vi "ClassPanel.vi"(8 "error in (no error)":errorcluster caption="entrée d'erreur (pas d'erreur)", 11 "AFG3102C.lvclass":refnum<class "AFG3102C.lvclass">) -> (0 "error out":errorcluster caption="sortie d'erreur", 3 "AFG3102C.lvclass Out":refnum<class "AFG3102C.lvclass">)   [LabVIEW 2019, in "AFG3102C.lvclass"]
uses:
  AFG3102C.lvclass
  C:/Programmes Labview/LabscanV1A/DevicesClass/BaseDevice/BaseDevice.lvclass
  BaseDevice/ClassQueueMess.ctl
  AFG3102C_Func.ctl
  AFG3102C.lvclass/AFG3102C.ctl
  BaseDevice/BaseDevice.lvclass/BaseDevice.ctl
  BaseDevice/Accessor/SetShowInstrNm.vi
  BaseDevice/Accessor/GetClassEvent.vi
  <userlib>/Tektronix AFG 3000 Series/Tektronix AFG 3000 Series.lvlib
panel:
  out "Trig":bool
  in  "Custom Impedance":dbl=400.0
  out "AcqTime":dbl caption="AcqTime(s)" format="%<%M:%S%5u>t"
  in  "Trig and wait":bool
  out "InitPulseLT_us_ch2":dbl=4.0 caption="InitPulseLT(us)" min=0.01 max=1000000000.0 step=0.01
  out "InitPulseHT_us_ch2":dbl=4.0 caption="InitPulseHT(us)" min=0.01 max=1000000000.0 step=0.01
  out "PulsePeriod_us_ch2":dbl=4.0 caption="Pulse Per ch2 (us)" min=0.01 max=1000000000.0 step=0.01
  in  "ForceTrig":bool
  in  "Output En 2":bool caption="Out2 En"
  in  "Out1 En":bool
  out "InitPulseLT_us":dbl=4.0 caption="InitPulseLT(us)" min=0.01 max=1000000000.0 step=0.01
  out "InitPulseHT_us":dbl=4.0 caption="InitPulseHT(us)" min=0.01 max=1000000000.0 step=0.01
  out "PulsePeriod_us":dbl=4.0 caption="Pulse Period (us)" min=0.01 max=1000000000.0 step=0.01
  in  "Con/Disc.":bool
  in  "Tk3102CTab":enum32{"MW Ch1", "Ch2 Laser", "Trig/Func"}(tab)
  in  "BefDel_us":dbl=0.15 caption="BeforeDelay(us)" min=0.0 max=1000000000.0 step=0.001
  in  "HighLevel(V)":dbl=5.0
  in  "LowLevel(V)":dbl
  in  "PLowTime_us":dbl=2.0 caption="Pulse Low\nTime(us)" min=0.01 max=1000000000.0 step=0.01
  in  "PulseCount":i32=30000 caption="Pulse count" min=0 step=1
  in  "BurstDel_us":dbl caption="BurstDelay(us)" min=0.0 max=1000000000.0 step=0.001
  in  "PHighTime_us":dbl=4.0 caption="Pulse High\nTime(us)" min=0.01 max=1000000000.0 step=0.01
  in  "OutputImp":u16(ring) caption="Output Impedance" items=["50 Ohm", "High Impedance", "Customized"]
  in  "AfterPulseDel(us)":dbl=0.1 caption="AfterPulseDelay(us)" min=0.01 max=1000000000.0 step=0.01
  in  "Link Ch":bool=TRUE
  in  "HighLevel(V)ch2":dbl=4.6 caption="HighLevel(V)"
  in  "LowLevel(V)ch2":dbl caption="LowLevel(V)"
  in  "PLowTime_us_ch2":dbl=2.0 caption="Pulse Low\nTime(us)" min=0.01 max=1000000000.0 step=0.01
  in  "PulseCount_ch2":i32=1 caption="Pulse count" min=0 step=1
  in  "PHighTime_us_ch2":dbl=10.0 caption="Pulse High\nTime(us)" min=0.01 max=1000000000.0 step=0.01
  in  "OutputImpch2":u16(ring)=2 caption="Output Impedance" items=["50 Ohm", "High Impedance", "Customized"]
  in  "BurstDel_us_ch2":dbl caption="Burst Delay ch2(us)" min=0.0 max=1000000000.0 step=0.001
  in  "Trigger Source":u16(ring)=1 items=["Internal"=3, "External"=1]
  in  "ExtTrigger Slope":u16(ring)=1 items=["Positive", "Negative"]
  in  "IntTriggRate(s)":dbl=1.0
  in  "Pulse Function":T1(ring)
  in  "Continuous2":bool caption="Continuous"
  out "ControlsNames":string[](array[string])
  in  "MainProgQ":refnum<queue>
  in  "MainProgQEvent":refnum<user-event>
  in  "Acq":bool
  in  "Stop":bool
  out "Init Program":bool
  # "Tek.AFG3102C"
  # "this MUST labeled with class name"
  # "this MUST be present and labeled \"Stop\" and \"Acq\""
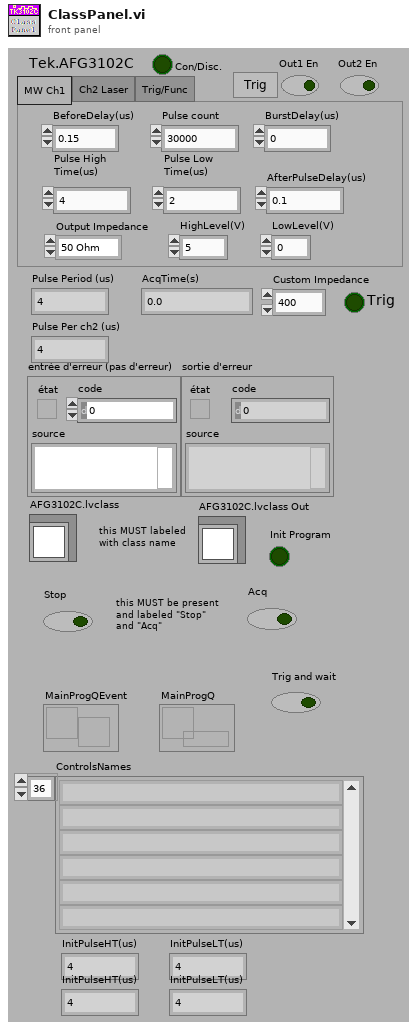
[diagram p1: front panel]
types:
  T1 = enum16{"Rabi", "Ramsey", "Ramsey Ext", "Rabi Ext Laser", "None"}
  T2 = typedef "AFG3102C.lvclass/AFG3102C_Func.ctl" = enum16{"RabiExt (Tau)", "Rabi (Tau)", "RamseyExt (Tau)", "Ramsey (Tau)"}
  T3 = enum16{"Enable", "Disable", "DisAndGrayed", "ReinitToDefVal", "EnumElementsArr"}
  T4 = typedef "ClassQueueMess.ctl" = u16
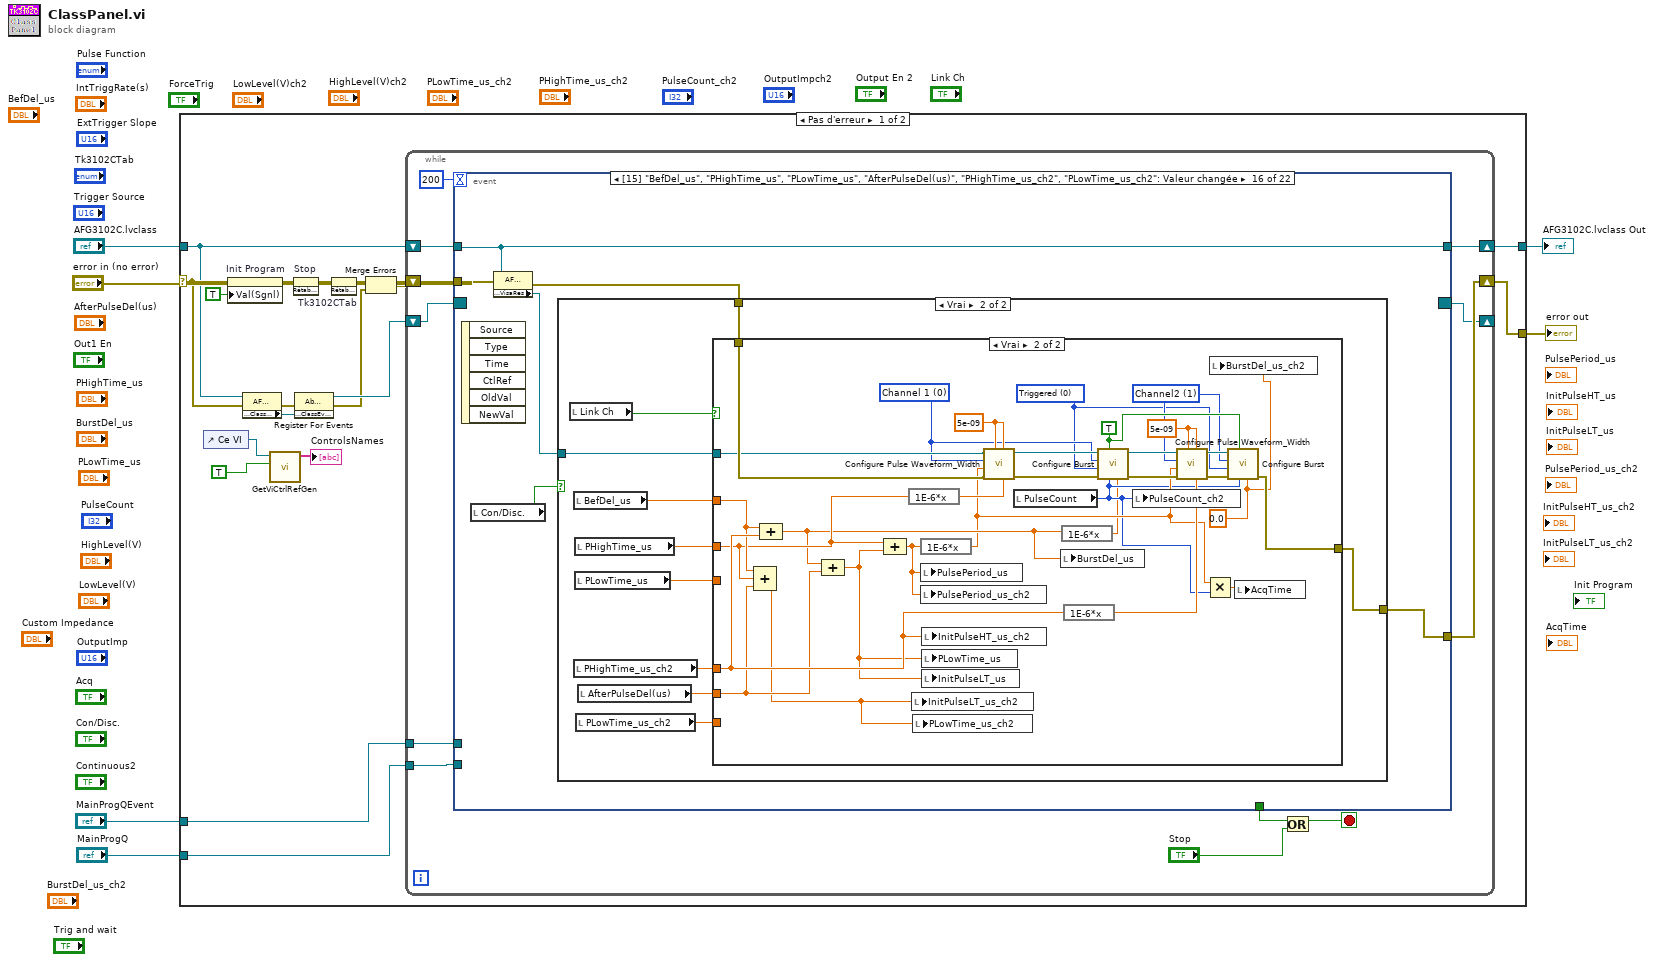
[diagram p0: block diagram]
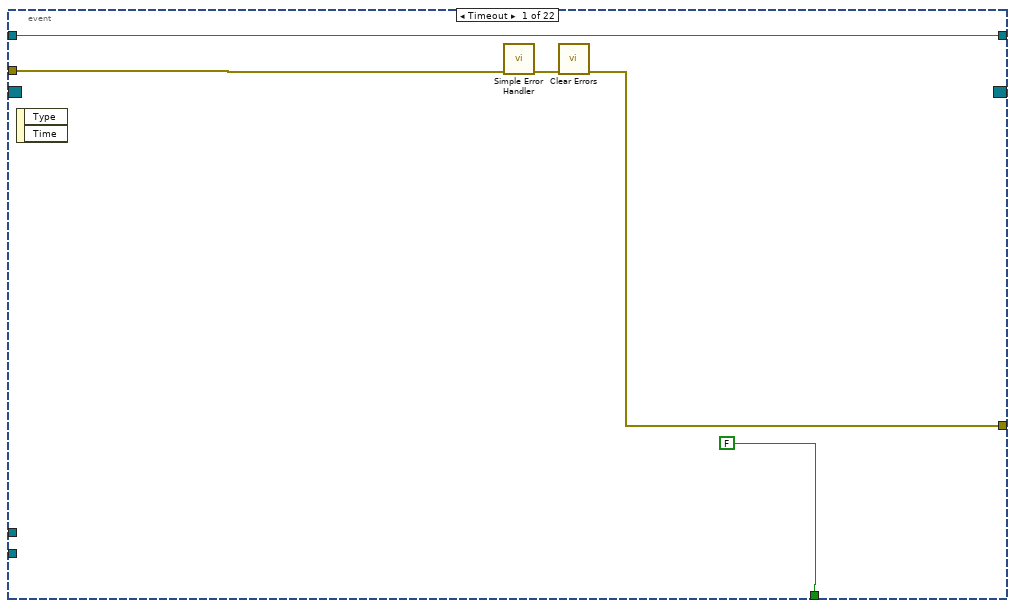
[diagram p2: hidden frame]
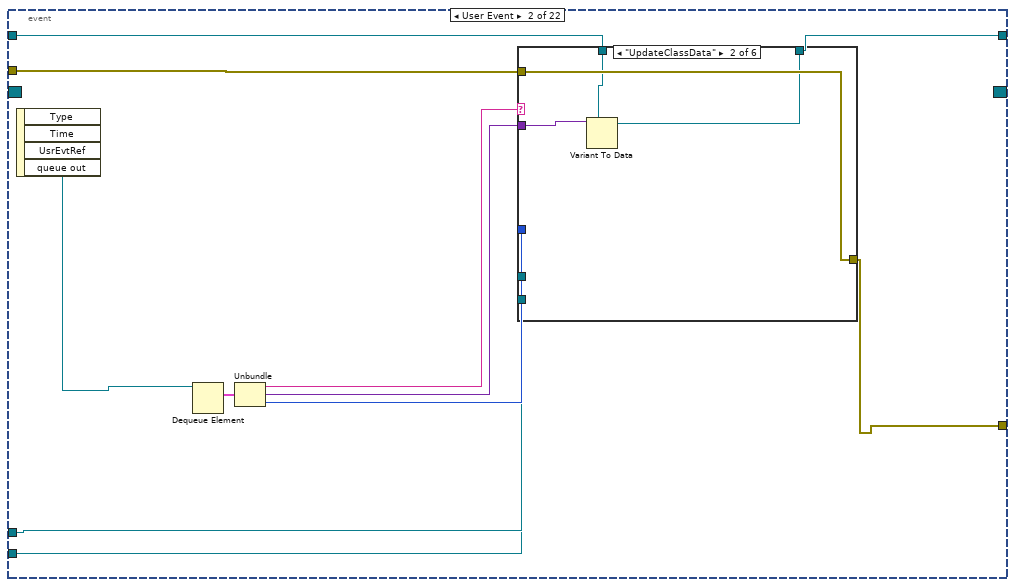
[diagram p3: hidden frame]
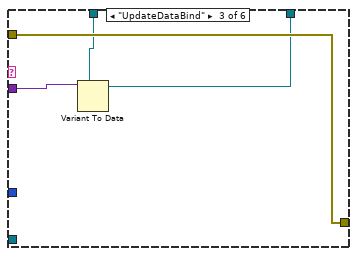
[diagram p5: hidden frame]
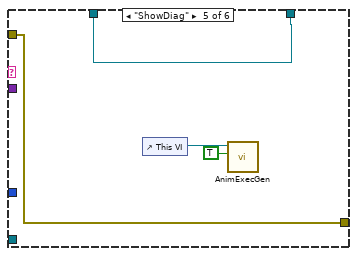
[diagram p7: hidden frame]
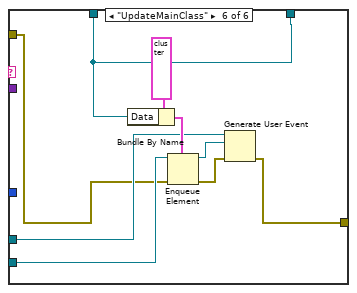
[diagram p8: hidden frame]
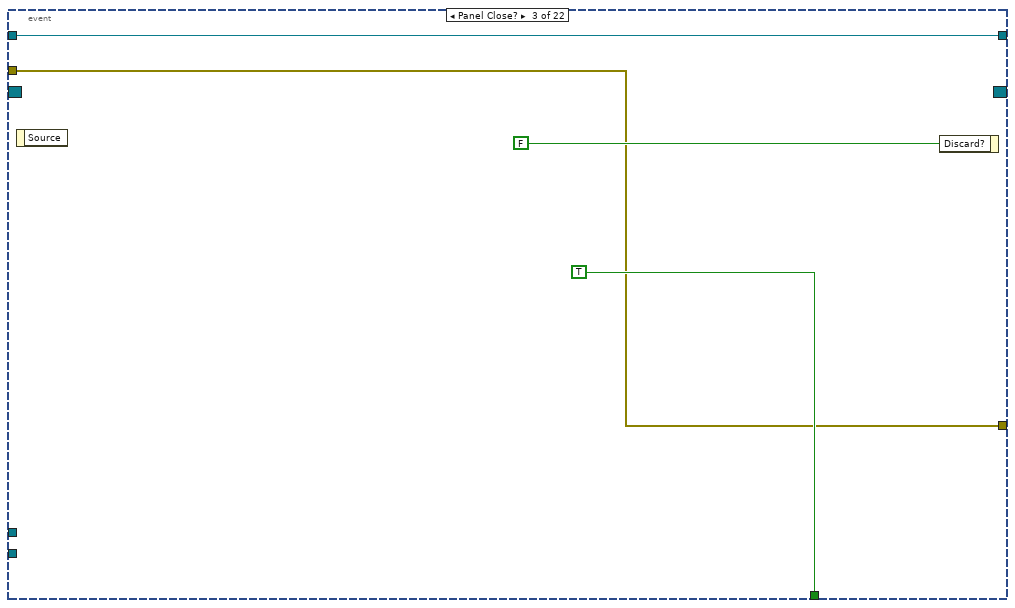
[diagram p9: hidden frame]
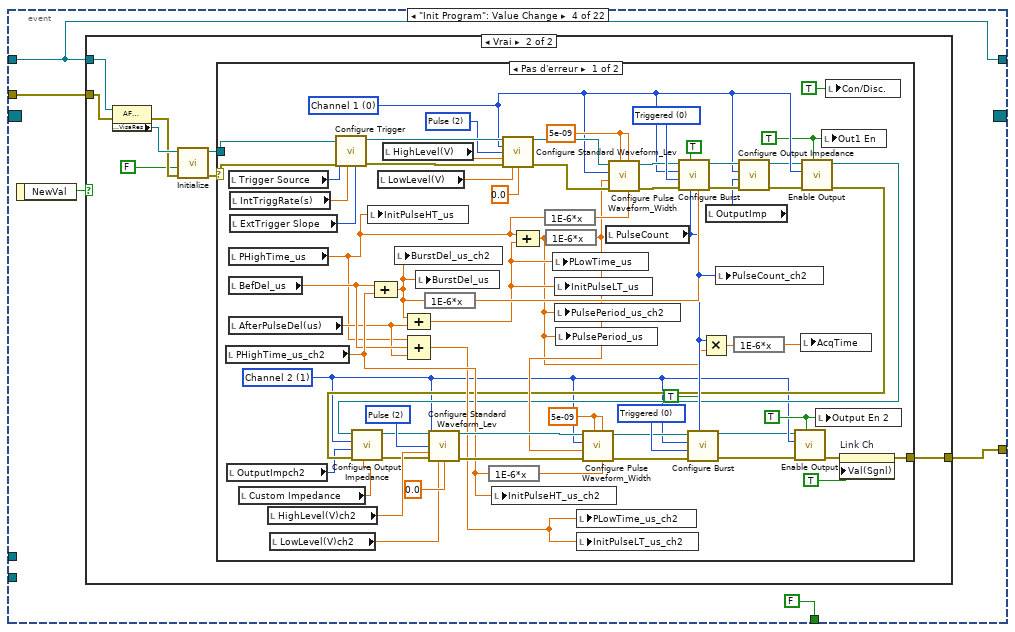
[diagram p10: hidden frame]
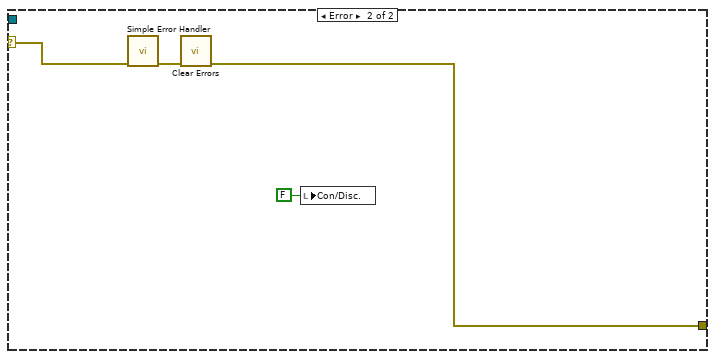
[diagram p12: hidden frame]
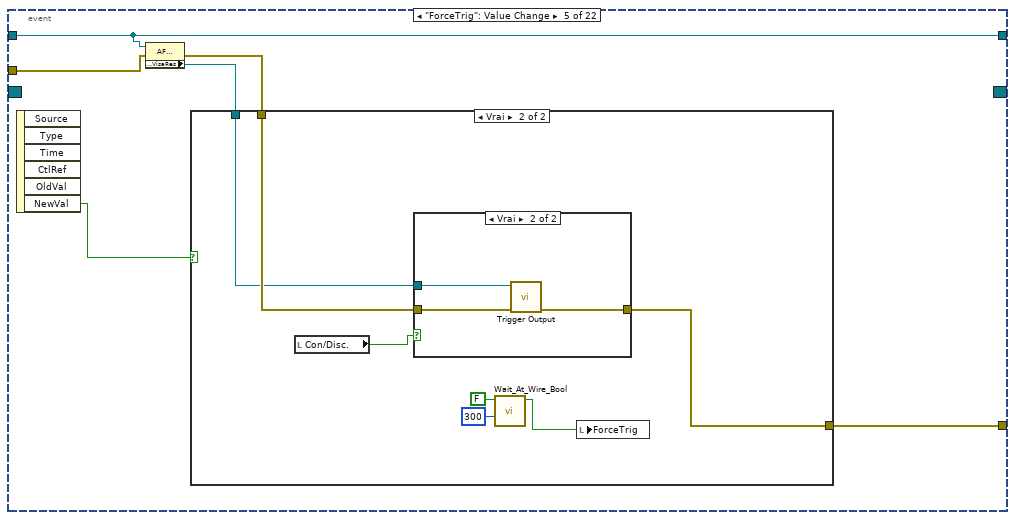
[diagram p13: hidden frame]
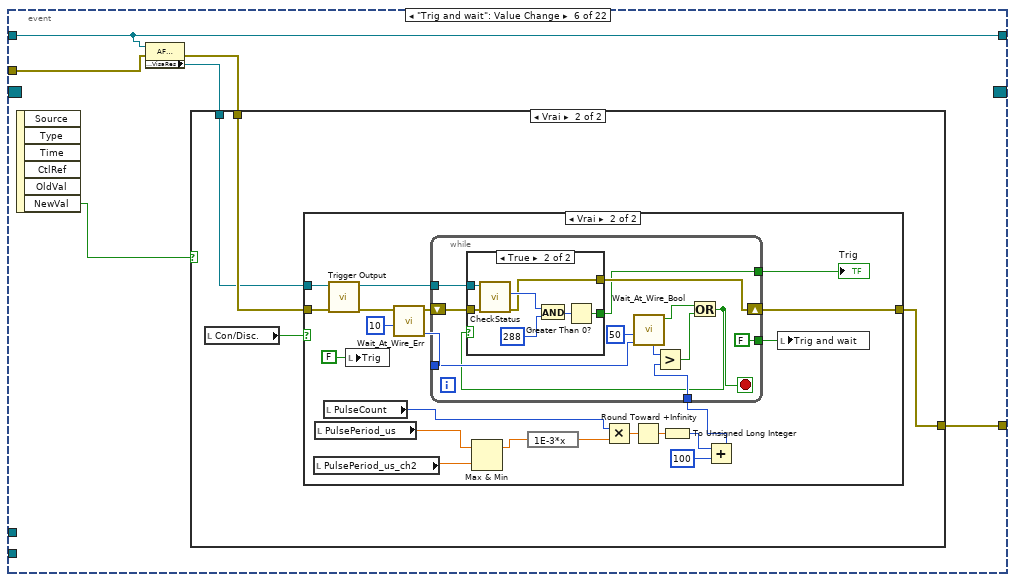
[diagram p16: hidden frame]
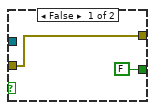
[diagram p19: hidden frame]
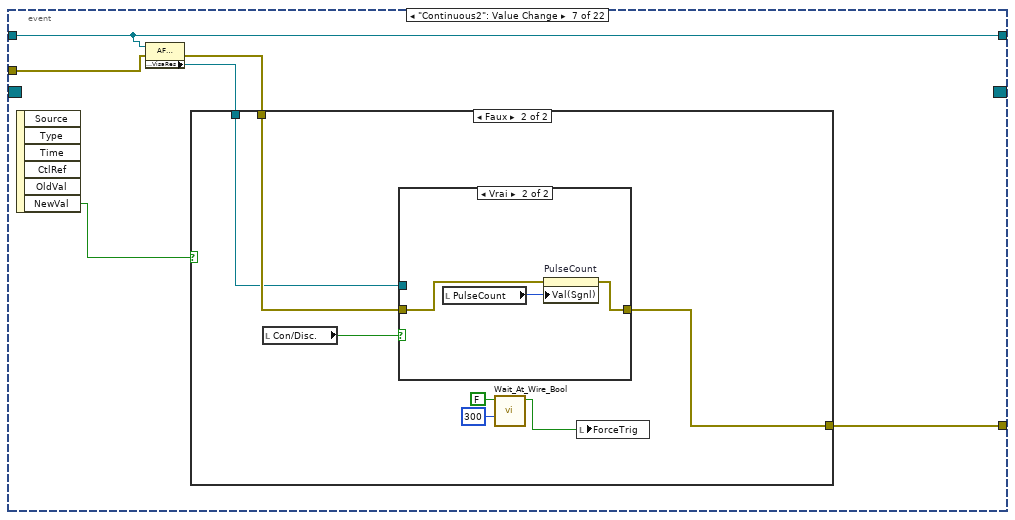
[diagram p20: hidden frame]
diagram:
  n1 = case shown="Pas d'erreur" "error in (no error)" {
    selector: "error in (no error)" -> [w7 w628]
    tunnel: [w24 w628] -> w5
    tunnel: "AFG3102C.lvclass" -> [w18 w627]
    tunnel: [w22 w627] -> w3
    tunnel: "MainProgQEvent" -> [w17 _]
    tunnel: "MainProgQ" -> [w16 _]
    frame No Error {
      n2 = control-ref of="Ce VI"() -> (w14:refnum<vi>)
      n3 = property on="Init Program" class="Bool (strict)"(error in=w7, "Val(Sgnl)"=TRUE ("Valeur (Signalisation)")) -> (error out=w21:errorcluster)  [unwired: 1 in, 1 out]
      n4 = property class="AFG3102C.lvclass"(reference=w18, error in=w7) -> (error out=w20:errorcluster, "Accessor:ClassEvent"=w19:refnum<user-event>)  [unwired: 1 out]
      n5 = call <userlib>:"GetViCtrlRefGen.vi"("InclTabCTrl"=TRUE, "VIRef"=w14) -> ("ControlsNames"=→"ControlsNames":string[])  [unwired: 7 in, 2 out]
      n6 = invoke on="Stop" class="Bool (strict)" method="RétablirValParDéfaut"(error in=w21) -> (error out=w12:errorcluster)  [unwired: 2 in, 2 out]
      n7 = register-events(error in=w20, w19) -> (reference out=w10:refnum<event-registration>, error out=w8:errorcluster)  [unwired: 1 in]
      n8 = invoke on="Tk3102CTab" class="Onglet (strict)" method="RétablirValParDéfaut"(error in=w12) -> (error out=w11:errorcluster)  [unwired: 2 in, 2 out]
      n9 = Merge Errors(w11, w8) -> (w9:errorcluster)
      n10 = while {
        shift-right: [w34] -> w24
        shift-left: w9 -> [w35]
        shift-right: [w31] -> w22
        shift-left: w18 -> [w33]
        shift-right: [w27] -> _
        shift-left: w10 -> [w28]
        tunnel: w17 -> [w26]
        tunnel: w16 -> [w25]
        stop <- w30 stop-if-true
        n11 = event shown="[15] \"BefDel_us\", \"PHighTime_us\", \"PLowTime_us\", \"AfterPulseDel(us)\", \"PHighTime_us_ch2\", \"PLowTime_us_ch2\": Valeur changée" {
          selector: w28 -> [_ _ _ _ _ _ _ _ _ _ _ _ _ _ _ _ _ _ _ _ _ _]
          dyn-events: [_ _ _ _ _ _ _ _ _ _ _ _ _ _ _ _ _ _ _ _ _ _] -> w27
          timeout: 200 -> [_ _ _ _ _ _ _ _ _ _ _ _ _ _ _ _ _ _ _ _ _ _]
          tunnel: w35 -> [w39 w51 w79 w85 w168 w187 w240 w282 w295 w303 w364 w384 w403 w417 w431 w477 w551 _ w576 w590 w604 w618]
          tunnel: [w37 w45 w79 w84 w165 w184 w237 w277 w290 w306 w359 w379 w399 w412 w426 w472 w553 _ w571 w585 w599 w613] -> w34
          tunnel: w33 -> [w40 w52 w78 w82 w169 w188 w241 w281 w294 w304 w363 w383 w405 w416 w430 w476 w550 w564 w575 w589 w603 w617]
          tunnel: [FALSE _ TRUE FALSE _ _ _ _ _ _ _ _ _ _ _ _ _ _ _ _ _ _] -> w32
          tunnel: [w40 w44 w78 w82 w169 w188 w241 w281 w294 w308 w363 w383 w404 w416 w430 w476 w550 w564 w575 w589 w603 w617] -> w31
          tunnel: w26 -> [_ w43 _ _ _ _ _ _ _ _ _ _ _ _ _ _ _ _ _ _ _ _]
          tunnel: w25 -> [_ w42 _ _ _ _ _ _ _ _ _ _ _ _ _ _ _ _ _ _ _ _]
          event Timeout {
            n12 = event-data() -> ()  [unwired: 1 in, 2 out]
            n13 = call <vilib>:"Simple Error Handler.vi"("error in (no error)"=w39) -> ("error out"=w38:errorcluster)  [unwired: 4 in, 4 out]
            n14 = call <vilib>:"Clear Errors.vi"("error in (no error)"=w38) -> ("error out"=w37:errorcluster)  [unwired: 5 in, 1 out]
          }
          event User Event {
            n15 = event-data() -> ("queue out"=w49:refnum<queue>)  [unwired: 1 in, 3 out]
            n16 = Dequeue Element(queue=w49) -> (element=w50:cluster{"Message":string, "Data":variant, i32})  [unwired: 2 in, 3 out]
            n17 = Unbundle(w50) -> ("Message"=w48:string, "Data"=w47:variant, w46:i32)
            n18 = case shown="\"UpdateClassData\"" w48 {
              tunnel: w51 -> [w54 w58 w62 w63 w67 w70]
              tunnel: w47 -> [_ w57 w61 _ _ _]
              tunnel: w52 -> [w53 w56 w60 w64 w68 w73]
              tunnel: [w53 w55 w59 w64 w68 w73] -> w44
              tunnel: [w54 w58 w62 w63 w67 w69] -> w45
              tunnel: w46 -> [_ _ _ _ _ _]
              tunnel: w43 -> [_ _ _ _ _ w72]
              tunnel: w42 -> [_ _ _ _ _ w71]
              frame Default {
              }
              frame "UpdateClassData" {
                n19 = Variant To Data(type=w56, Variant=w57) -> (data=w55:refnum<class "AFG3102C.lvclass">)  [unwired: 1 in, 1 out]
              }
              frame "UpdateDataBind" {
                n20 = Variant To Data(type=w60, Variant=w61) -> (data=w59:refnum<class "AFG3102C.lvclass">)  [unwired: 1 in, 1 out]
              }
              frame "MeasDone" {
              }
              frame "ShowDiag" {
                n21 = control-ref of="This VI"() -> (w66:refnum<vi>)
                n22 = call <userlib>:"AnimExecGen.vi"("Animer l'exécution ?"=TRUE, "ViRef"=w66) -> ()  [unwired: 9 in, 1 out]
              }
              frame "UpdateMainClass" {
                n23 = Bundle By Name(cluster=cluster{"Message":string, "Data":variant, i32} {"Message"="", "Data"=variant, 0} ("élément"), "Data"=w73) -> (w74:cluster{"Message":string, "Data":variant, i32})
                n24 = Enqueue Element(queue=w71, element=w74, error in (no error)=w70) -> (queue out=w77:refnum<queue>, error out=w76:errorcluster)  [unwired: 1 in, 1 out]
                n25 = Generate User Event(user event=w72, event data cluster=w77, error in=w76) -> (error out=w69:errorcluster)  [unwired: 1 in, 1 out]
              }
            }
          }
          event Panel Close? {
            n26 = event-data() -> ()  [unwired: 1 in, 1 out]
            n27 = event-data("Discard?"=FALSE ("Rejeter ?")) -> ()  [unwired: 1 in, 1 out]
          }
          event "Init Program": Value Change {
            n28 = event-data() -> ("NewVal"=w86:bool)  [unwired: 1 in]
            n29 = case shown="Vrai" w86 {
              tunnel: w85 -> [w87 w95]
              tunnel: [w87 w89] -> w84
              tunnel: w82 -> [_ w88]
              frame False {
              }
              frame True {
                n30 = property class="AFG3102C.lvclass"(reference=w88, error in=w95) -> (error out=w93:errorcluster, "Accessor:VisaRes"=w94:refnum<visa-resource-name>)  [unwired: 1 out]
                n31 = call <userlib>:"Initialize.vi"("error in (no error)"=w93, "Reset (True)"=FALSE, "VISA resource name"=w94) -> ("error out"=w90:errorcluster, "VISA resource name out"=w91:refnum<visa-resource-name>)  [unwired: 7 in]
                n32 = case shown="Pas d'erreur" w90 {
                  selector: w90 -> [w145 w164]
                  tunnel: w91 -> [w159 _]
                  tunnel: [w113 w162] -> w89
                  frame No Error {
                    w123 = TRUE ("Enable Output (T: Enable)")
                    w127 = u16 0 items=["Triggered", "Gated"] ("Burst Mode (0: Triggered)")
                    w131 = 5e-09 ("Leading Edge Time (5.0E-8)")
                    w101 = u16 1 items=["Channel 1", "Channel 2"] ("Channel (0: Channel 1)")
                    w133 = u16 2 items=["Sine", "Square", "Pulse", "Ramp", "Noise", "DC", "Sin(x)/x", "Gaussian", "Lorentz", "Exponential Rise", "Exponential Decay", "Haversine"] ("Waveform Function (0: Sine)")
                    w140 = TRUE ("Enable Output (T: Enable)")
                    w151 = u16 2 items=["Sine", "Square", "Pulse", "Ramp", "Noise", "DC", "Sin(x)/x", "Gaussian", "Lorentz", "Exponential Rise", "Exponential Decay", "Haversine"] ("Waveform Function (0: Sine)")
                    w155 = 5e-09 ("Leading Edge Time (5.0E-8)")
                    w158 = u16 0 items=["Triggered", "Gated"] ("Burst Mode (0: Triggered)")
                    w143 = u16 0 items=["Channel 1", "Channel 2"] ("Channel (0: Channel 1)")
                    n33 = local read "PHighTime_us_ch2"() -> (w118:dbl)
                    n34 = local read "OutputImpch2"() -> (w100:u16)
                    n35 = local read "Trigger Source"() -> (w139:u16)
                    n36 = local read "PHighTime_us"() -> (w110:dbl)
                    n37 = local read "BefDel_us"() -> (w117:dbl)
                    n38 = local read "AfterPulseDel(us)"() -> (w116:dbl)
                    n39 = local read "IntTriggRate(s)"() -> (w137:dbl)
                    n40 = local read "ExtTrigger Slope"() -> (w138:u16)
                    n41 = local read "Custom Impedance"() -> (w99:dbl)
                    n42 = local read "HighLevel(V)ch2"() -> (w134:dbl)
                    n43 = local read "LowLevel(V)ch2"() -> (w135:dbl)
                    n44 = call <userlib>:"Configure Trigger.vi"("External Trigger Slope (0: Positive)"=w138, "Internal Trigger Rate (500)"=w137, "error in (no error)"=w145, "Trigger Source (3:Internal)"=w139, "VISA resource name"=w159) -> ("error out"=w150:errorcluster, "VISA resource name out"=w153:refnum<visa-resource-name>)  [unwired: 5 in]
                    n45 = local write "InitPulseHT_us"(w110) -> ()
                    n46 = Compound Arithmetic op=ADD(w117, w118) -> (w111:dbl)
                    n47 = local read "LowLevel(V)"() -> (w149:dbl)
                    n48 = local read "HighLevel(V)"() -> (w125:dbl)
                    n49 = local write "BurstDel_us_ch2"(w111) -> ()
                    n50 = Compound Arithmetic op=ADD(w111, w116) -> (w120:dbl)
                    n51 = Compound Arithmetic op=ADD(w110, w117, w116) -> (w115:dbl)
                    n52 = local write "BurstDel_us"(w111) -> ()
                    n53 = expression code="1E-6*x"(w111) -> (w122:dbl)
                    n54 = expression code="1E-6*x"(w118) -> (w124:dbl)
                    n55 = local write "InitPulseHT_us_ch2"(w118) -> ()
                    n56 = call <userlib>:"Configure Standard Waveform_Lev.vi"("VISA resource name"=w153, "Channel (0: Channel 1)"=w143, "Waveform Function (0: Sine)"=w151, "HighLevel (V)"=w125, "error in (no error)"=w150, "LowLevel (V)"=w149, "Phase Level (-1)"=0.0) -> ("VISA resource name out"=w152:refnum<visa-resource-name>, "error out"=w154:errorcluster)  [unwired: 7 in]
                    n57 = Compound Arithmetic op=ADD(w110, w120) -> (w108:dbl)
                    n58 = expression code="1E-6*x"(w110) -> (w121:dbl)
                    n59 = expression code="1E-6*x"(w108) -> (w119:dbl)
                    n60 = local write "PLowTime_us"(w120) -> ()
                    n61 = local write "InitPulseLT_us"(w120) -> ()
                    n62 = local write "PulsePeriod_us_ch2"(w108) -> ()
                    n63 = local write "PulsePeriod_us"(w108) -> ()
                    n64 = local write "PLowTime_us_ch2"(w115) -> ()
                    n65 = local write "InitPulseLT_us_ch2"(w115) -> ()
                    n66 = local read "PulseCount"() -> (w109:i32)
                    n67 = call <userlib>:"Configure Pulse Waveform_Width.vi"("Width(s)"=w121, "Trailing Edge Time (5.0E-8)"=w155, "Leading Edge Time (5.0E-8)"=w155, "error in (no error)"=w154, "Period(s)"=w119, "Channel (0: Channel 1)"=w143, "VISA resource name"=w152) -> ("error out"=w157:errorcluster, "VISA resource name out"=w156:refnum<visa-resource-name>)  [unwired: 3 in]
                    n68 = call <userlib>:"Configure Burst.vi"("Busrt Delay  (0.0s)"=w122, "Burst Count (5)"=w109, "Enable Burst (T: Enable)"=TRUE ("Enable Burst"), "error in (no error)"=w157, "Burst Mode (0: Triggered)"=w158, "Channel (0: Channel 1)"=w143, "VISA resource name"=w156) -> ("error out"=w148:errorcluster, "VISA resource name out"=w147:refnum<visa-resource-name>)  [unwired: 3 in]
                    n69 = Multiply(x=w109, y=w108) -> (x*y=w107:dbl)
                    n70 = local read "OutputImp"() -> (w146:u16)
                    n71 = local write "PulseCount_ch2"(w109) -> ()
                    n72 = expression code="1E-6*x"(w107) -> (w106:dbl)
                    n73 = call <userlib>:"Configure Output Impedance.vi"("error in (no error)"=w148, "Impedance (0: 50 Ohm)"=w146, "Channel (0: Channel 1)"=w143, "VISA resource name"=w147) -> ("error out"=w144:errorcluster, "VISA resource name out"=w142:refnum<visa-resource-name>)  [unwired: 6 in]
                    n74 = local write "AcqTime"(w106) -> ()
                    n75 = call <userlib>:"Enable Output.vi"("Enable Output (T: Enable)"=w140, "error in (no error)"=w144, "Channel (0: Channel 1)"=w143, "VISA resource name"=w142) -> ("error out"=w102:errorcluster, "VISA resource name out"=w103:refnum<visa-resource-name>)  [unwired: 5 in]
                    n76 = call <userlib>:"Configure Output Impedance.vi"("Customized Impedance (50.0 Ohm)"=w99, "error in (no error)"=w102, "Impedance (0: 50 Ohm)"=w100, "Channel (0: Channel 1)"=w101, "VISA resource name"=w103) -> ("error out"=w105:errorcluster, "VISA resource name out"=w104:refnum<visa-resource-name>)  [unwired: 5 in]
                    n77 = call <userlib>:"Configure Standard Waveform_Lev.vi"("VISA resource name"=w104, "Channel (0: Channel 1)"=w101, "Waveform Function (0: Sine)"=w133, "HighLevel (V)"=w134, "error in (no error)"=w105, "LowLevel (V)"=w135, "Phase Level (-1)"=0.0) -> ("VISA resource name out"=w130:refnum<visa-resource-name>, "error out"=w129:errorcluster)  [unwired: 7 in]
                    n78 = call <userlib>:"Configure Pulse Waveform_Width.vi"("Width(s)"=w124, "Trailing Edge Time (5.0E-8)"=w131, "Leading Edge Time (5.0E-8)"=w131, "error in (no error)"=w129, "Period(s)"=w119, "Channel (0: Channel 1)"=w101, "VISA resource name"=w130) -> ("error out"=w128:errorcluster, "VISA resource name out"=w126:refnum<visa-resource-name>)  [unwired: 3 in]
                    n79 = call <userlib>:"Configure Burst.vi"("Burst Count (5)"=w109, "Enable Burst (T: Enable)"=TRUE, "error in (no error)"=w128, "Burst Mode (0: Triggered)"=w127, "Channel (0: Channel 1)"=w101, "VISA resource name"=w126) -> ("error out"=w98:errorcluster, "VISA resource name out"=w97:refnum<visa-resource-name>)  [unwired: 4 in]
                    n80 = call <userlib>:"Enable Output.vi"("Enable Output (T: Enable)"=w123, "error in (no error)"=w98, "Channel (0: Channel 1)"=w101, "VISA resource name"=w97) -> ("error out"=w114:errorcluster)  [unwired: 5 in, 1 out]
                    n81 = local write "Output En 2"(w123) -> ()
                    n82 = local write "Out1 En"(w140) -> ()
                    n83 = local write "Con/Disc."(TRUE ("Con/Disc.")) -> ()
                    n84 = property on="Link Ch" class="Bool (strict)"(error in=w114, "Val(Sgnl)"=TRUE ("Valeur (Signalisation)")) -> (error out=w113:errorcluster)  [unwired: 1 in, 1 out]
                  }
                  frame Error {
                    n85 = call <vilib>:"Simple Error Handler.vi"("error in (no error)"=w164) -> ("error out"=w163:errorcluster)  [unwired: 4 in, 4 out]
                    n86 = call <vilib>:"Clear Errors.vi"("error in (no error)"=w163) -> ("error out"=w162:errorcluster)  [unwired: 5 in, 1 out]
                    n87 = local write "Con/Disc."(FALSE ("Con/Disc.")) -> ()
                  }
                }
              }
            }
          }
          event "ForceTrig": Value Change {
            n88 = event-data() -> ("NewVal"=w170:bool)  [unwired: 1 in, 5 out]
            n89 = property class="AFG3102C.lvclass"(reference=w169, error in=w168) -> (error out=w167:errorcluster, "Accessor:VisaRes"=w166:refnum<visa-resource-name>)  [unwired: 1 out]
            n90 = case shown="Vrai" w170 {
              tunnel: w167 -> [w171 w175]
              tunnel: w166 -> [_ w174]
              tunnel: [w171 w173] -> w165
              frame False {
              }
              frame True {
                n91 = local read "Con/Disc."() -> (w172:bool)
                n92 = case shown="Vrai" w172 {
                  tunnel: w175 -> [w179 w182]
                  tunnel: w174 -> [_ w181]
                  tunnel: [w179 w180] -> w173
                  frame False {
                  }
                  frame True {
                    n93 = call <userlib>:"Trigger Output.vi"("error in (no error)"=w182, "VISA resource name"=w181) -> ("error out"=w180:errorcluster)  [unwired: 7 in, 1 out]
                  }
                }
                n94 = call <userlib>:"Wait_At_Wire_Bool.vi"("Wait (ms)"=u32 300, "error in (no error)"=FALSE) -> ("error out"=w178:bool)  [unwired: 7 in, 2 out]
                n95 = local write "ForceTrig"(w178) -> ()
              }
            }
          }
          event "Trig and wait": Value Change {
            n96 = event-data() -> ("NewVal"=w183:bool)  [unwired: 1 in, 5 out]
            n97 = property class="AFG3102C.lvclass"(reference=w188, error in=w187) -> (error out=w186:errorcluster, "Accessor:VisaRes"=w185:refnum<visa-resource-name>)  [unwired: 1 out]
            n98 = case shown="Vrai" w183 {
              tunnel: w186 -> [w189 w193]
              tunnel: w185 -> [_ w192]
              tunnel: [w189 w191] -> w184
              frame False {
              }
              frame True {
                n99 = local read "Con/Disc."() -> (w190:bool)
                n100 = case shown="Vrai" w190 {
                  tunnel: w193 -> [w194 w215]
                  tunnel: w192 -> [_ w214]
                  tunnel: [w194 w210] -> w191
                  frame False {
                  }
                  frame True {
                    n101 = local read "PulsePeriod_us_ch2"() -> (w212:dbl)
                    n102 = local read "PulsePeriod_us"() -> (w213:dbl)
                    n103 = local read "PulseCount"() -> (w202:i32)
                    n104 = call <userlib>:"Trigger Output.vi"("error in (no error)"=w215, "VISA resource name"=w214) -> ("error out"=w207:errorcluster, "VISA resource name out"=w211:refnum<visa-resource-name>)  [unwired: 7 in]
                    n105 = local write "Trig"(FALSE ("Trig")) -> ()
                    n106 = call <userlib>:"Wait_At_Wire_Err.vi"("Wait (ms)"=u32 10, "error in (no error)"=w207) -> ("Clock(ms)"=w205:u32, "error out"=w206:errorcluster)  [unwired: 7 in, 1 out]
                    n107 = Max & Min(x=w213, y=w212) -> (max(x,y)=w209:dbl)  [unwired: 1 out]
                    n108 = expression code="1E-3*x"(w209) -> (w203:dbl)
                    n109 = Multiply(x=w202, y=w203) -> (x*y=w201:dbl)
                    n110 = Round Toward +Infinity(x=w201) -> (ceil(x): smallest int >= x=w200:dbl)
                    n111 = To Unsigned Long Integer(number=w200) -> (unsigned 32bit integer=w198:u32)
                    n112 = Add(x=w198, y=u32 100) -> (x+y=w199:u32)
                    n113 = while {
                      tunnel: w211 -> [w226]
                      tunnel: w205 -> [w223]
                      shift-right: [w225] -> w210
                      shift-left: w206 -> [w227]
                      tunnel: w199 -> [w221]
                      tunnel: [FALSE ("Trig and wait")] -> w208
                      tunnel: [w216] -> w195
                      stop <- w217 stop-if-true
                      n114 = call <userlib>:"Wait_At_Wire_Bool.vi"("InitClock(ms)"=w223, "Wait (ms)"=u32 50) -> ("error out"=w224:bool, "Delta(ms)"=w222:u32)  [unwired: 7 in, 1 out]
                      n115 = Greater?(x=w222, y=w221) -> (0:w220:bool)
                      n116 = Or(x=w224, y=w220) -> (x .or. y?=w217:bool)
                      n117 = case shown="Faux" w217 {
                        tunnel: w227 -> [w229 w236]
                        tunnel: w226 -> [_ w235]
                        tunnel: [w229 w231] -> w225
                        tunnel: [FALSE w230] -> w216
                        frame False {
                        }
                        frame True {
                          n118 = call <userlib>:"CheckStatus.vi"("error in (no error)"=w236, "VISA resource name"=w235) -> ("error out"=w231:errorcluster, "Oper Status"=w234:u16)  [unwired: 4 in, 4 out]
                          n119 = And(x=w234, y=u16 288) -> (x .and. y?=w232:u16)
                          n120 = Greater Than 0?(x=w232) -> (x > 0?=w230:bool)
                        }
                      }
                    }
                    "Trig" <- w195
                    n121 = local write "Trig and wait"(w208) -> ()
                  }
                }
              }
            }
          }
          event "Continuous2": Value Change {
            n122 = event-data() -> ("NewVal"=w242:bool)  [unwired: 1 in, 5 out]
            n123 = property class="AFG3102C.lvclass"(reference=w241, error in=w240) -> (error out=w239:errorcluster, "Accessor:VisaRes"=w238:refnum<visa-resource-name>)  [unwired: 1 out]
            n124 = case shown="Faux" w242 {
              tunnel: w239 -> [w246 w269]
              tunnel: w238 -> [w245 w268]
              tunnel: [w244 w267] -> w237
              frame True {
                n125 = local read "Con/Disc."() -> (w243:bool)
                n126 = case shown="Vrai" w243 {
                  tunnel: w246 -> [w250 w265]
                  tunnel: w245 -> [_ w264]
                  tunnel: [w250 w251] -> w244
                  frame False {
                  }
                  frame True {
                    w259 = u16 1 items=["Channel 1", "Channel 2"] ("Channel (0: Channel 1)")
                    w261 = TRUE ("Burst Cont")
                    w258 = u16 0 items=["Triggered", "Gated"] ("Burst Mode (0: Triggered)")
                    w263 = u16 0 items=["Channel 1", "Channel 2"] ("Channel (0: Channel 1)")
                    n127 = local read "BurstDel_us"() -> (w254:dbl)
                    n128 = local read "Link Ch"() -> (w257:bool)
                    n129 = Select(t=w254, s=w257, f=0.0 ("cas faux")) -> (s? t:f=w256:dbl)
                    n130 = call <userlib>:"Configure Burst.vi"("Busrt Delay  (0.0s)"=w256, "Burst Cont"=w261, "error in (no error)"=w265, "Burst Mode (0: Triggered)"=w258, "Channel (0: Channel 1)"=w263, "VISA resource name"=w264) -> ("error out"=w262:errorcluster, "VISA resource name out"=w260:refnum<visa-resource-name>)  [unwired: 4 in]
                    n131 = call <userlib>:"Configure Burst.vi"("Burst Cont"=w261, "error in (no error)"=w262, "Burst Mode (0: Triggered)"=w258, "Channel (0: Channel 1)"=w259, "VISA resource name"=w260) -> ("error out"=w253:errorcluster, "VISA resource name out"=w252:refnum<visa-resource-name>)  [unwired: 5 in]
                    n132 = call <userlib>:"Trigger Output.vi"("error in (no error)"=w253, "VISA resource name"=w252) -> ("error out"=w251:errorcluster)  [unwired: 7 in, 1 out]
                  }
                }
                n133 = call <userlib>:"Wait_At_Wire_Bool.vi"("Wait (ms)"=u32 300, "error in (no error)"=FALSE) -> ("error out"=w249:bool)  [unwired: 7 in, 2 out]
                n134 = local write "ForceTrig"(w249) -> ()
              }
              frame False {
                n135 = local read "Con/Disc."() -> (w266:bool)
                n136 = case shown="Vrai" w266 {
                  tunnel: w269 -> [w273 w276]
                  tunnel: w268 -> [_ _]
                  tunnel: [w273 w275] -> w267
                  frame False {
                  }
                  frame True {
                    n137 = local read "PulseCount"() -> (w274:i32)
                    n138 = property on="PulseCount" class="NumNb (strict)"(error in=w276, "Val(Sgnl)"=w274) -> (error out=w275:errorcluster)  [unwired: 1 in, 1 out]
                  }
                }
                n139 = call <userlib>:"Wait_At_Wire_Bool.vi"("Wait (ms)"=u32 300, "error in (no error)"=FALSE) -> ("error out"=w272:bool)  [unwired: 7 in, 2 out]
                n140 = local write "ForceTrig"(w272) -> ()
              }
            }
          }
          event "Out1 En": Value Change {
            n141 = event-data() -> ("NewVal"=w283:bool)  [unwired: 1 in, 5 out]
            n142 = local read "Con/Disc."() -> (w279:bool)
            n143 = property class="AFG3102C.lvclass"(reference=w281, error in=w282) -> (error out=w278:errorcluster, "Accessor:VisaRes"=w280:refnum<visa-resource-name>)  [unwired: 1 out]
            n144 = case shown="Vrai" w279 {
              tunnel: w283 -> [_ w289]
              tunnel: w280 -> [_ w288]
              tunnel: w278 -> [w284 w287]
              tunnel: [w284 w286] -> w277
              frame False {
              }
              frame True {
                w285 = u16 0 items=["Channel 1", "Channel2"] ("Channel (0: Channel 1)")
                n145 = call <userlib>:"Enable Output.vi"("Enable Output (T: Enable)"=w289, "error in (no error)"=w287, "Channel (0: Channel 1)"=w285, "VISA resource name"=w288) -> ("error out"=w286:errorcluster)  [unwired: 5 in, 1 out]
              }
            }
          }
          event "Output En 2": Value Change {
            n146 = event-data() -> ("NewVal"=w296:bool)  [unwired: 1 in, 5 out]
            n147 = local read "Con/Disc."() -> (w292:bool)
            n148 = property class="AFG3102C.lvclass"(reference=w294, error in=w295) -> (error out=w291:errorcluster, "Accessor:VisaRes"=w293:refnum<visa-resource-name>)  [unwired: 1 out]
            n149 = case shown="Vrai" w292 {
              tunnel: w296 -> [_ w302]
              tunnel: w293 -> [_ w301]
              tunnel: w291 -> [w297 w300]
              tunnel: [w297 w299] -> w290
              frame False {
              }
              frame True {
                w298 = u16 1 items=["Channel 1", "Channel2"] ("Channel (0: Channel 1)")
                n150 = call <userlib>:"Enable Output.vi"("Enable Output (T: Enable)"=w302, "error in (no error)"=w300, "Channel (0: Channel 1)"=w298, "VISA resource name"=w301) -> ("error out"=w299:errorcluster)  [unwired: 5 in, 1 out]
              }
            }
          }
          event "Pulse Function": Value Change {
            w305 = T4 1 items=["UpdateClassData", "UpdateMainClass", "UpdateDataBind", "ReInitDevice", "Custom", "ClosePan"] ("Menu déroulant")
            n151 = event-data() -> ("NewVal"=w310:T1)  [unwired: 1 in, 5 out]
            n152 = case shown="\"Ramsey Ext\"" w310 {
              tunnel: [w322 w334 w346 w358] -> w309
              tunnel: w304 -> [w313 w325 w337 w349]
              tunnel: [w321 w333 w345 w357] -> w307
              tunnel: w303 -> [w311 w323 w335 w350]
              frame "Rabi", Default {
                w315 = string[] [] ("SubDatDisplayNm")
                w317 = string[] ["RabiDelay(Tau)"]
                n153 = Bundle By Name(cluster=w313, "Functions"=AFG3102C_Func."Rabi (Tau)") -> (w312:refnum<class "AFG3102C.lvclass">)
                n154 = Array Size(array=w317) -> (size(s)=w320:i32)
                n155 = Initialize Array(TRUE, w320) -> (w318:bool[])
                n156 = property class="AFG3102C.lvclass"(reference=w312, error in=w311, "Accessor:SubDatDisplayNm"=w315, "Accessor:SubScanTable(y)"=dbl[] [] ("SubScanTable(y)"), "Accessor:ArrayDatNm"=w317, "Accessor:DataNames"=w315, "Accessor:SubVarParNm X"=w315, "Accessor:SubVarParNm Y"=w315, "Accessor:DatDisplayNm"=w315, "Accessor:ShowInstrNm"=w318) -> (reference out=w322:refnum<class "AFG3102C.lvclass">, error out=w321:errorcluster)
              }
              frame "Ramsey Ext" {
                w327 = string[] [] ("SubDatDisplayNm")
                w329 = string[] ["RamseyExt(Tau)"]
                n157 = Bundle By Name(cluster=w325, "Functions"=AFG3102C_Func."RamseyExt (Tau)") -> (w324:refnum<class "AFG3102C.lvclass">)
                n158 = Array Size(array=w329) -> (size(s)=w332:i32)
                n159 = Initialize Array(TRUE, w332) -> (w330:bool[])
                n160 = property class="AFG3102C.lvclass"(reference=w324, error in=w323, "Accessor:SubDatDisplayNm"=w327, "Accessor:SubScanTable(y)"=dbl[] [] ("SubScanTable(y)"), "Accessor:ArrayDatNm"=w329, "Accessor:DataNames"=w327, "Accessor:SubVarParNm X"=w327, "Accessor:SubVarParNm Y"=w327, "Accessor:DatDisplayNm"=w327, "Accessor:ShowInstrNm"=w330) -> (reference out=w334:refnum<class "AFG3102C.lvclass">, error out=w333:errorcluster)
              }
              frame "Rabi Ext Laser" {
                w339 = string[] [] ("SubDatDisplayNm")
                w341 = string[] ["RabiExt(Tau)"]
                n161 = Bundle By Name(cluster=w337, "Functions"=AFG3102C_Func."RabiExt (Tau)") -> (w336:refnum<class "AFG3102C.lvclass">)
                n162 = Array Size(array=w341) -> (size(s)=w344:i32)
                n163 = Initialize Array(TRUE, w344) -> (w342:bool[])
                n164 = property class="AFG3102C.lvclass"(reference=w336, error in=w335, "Accessor:SubDatDisplayNm"=w339, "Accessor:SubScanTable(y)"=dbl[] [] ("SubScanTable(y)"), "Accessor:ArrayDatNm"=w341, "Accessor:DataNames"=w339, "Accessor:SubVarParNm X"=w339, "Accessor:SubVarParNm Y"=w339, "Accessor:DatDisplayNm"=w339, "Accessor:ShowInstrNm"=w342) -> (reference out=w346:refnum<class "AFG3102C.lvclass">, error out=w345:errorcluster)
              }
              frame "Ramsey" {
                w351 = string[] ["RamseyDelay(Tau)"]
                w355 = string[] [] ("SubDatDisplayNm")
                n165 = Bundle By Name(cluster=w349, "Functions"=AFG3102C_Func."Ramsey (Tau)") -> (w348:refnum<class "AFG3102C.lvclass">)
                n166 = Array Size(array=w351) -> (size(s)=w354:i32)
                n167 = Initialize Array(TRUE, w354) -> (w352:bool[])
                n168 = property class="AFG3102C.lvclass"(reference=w348, error in=w350, "Accessor:SubDatDisplayNm"=w355, "Accessor:SubScanTable(y)"=dbl[] [] ("SubScanTable(y)"), "Accessor:ArrayDatNm"=w355, "Accessor:DataNames"=w351, "Accessor:SubVarParNm X"=w355, "Accessor:SubVarParNm Y"=w355, "Accessor:DatDisplayNm"=w355, "Accessor:ShowInstrNm"=w352) -> (reference out=w358:refnum<class "AFG3102C.lvclass">, error out=w357:errorcluster)
              }
            }
            n169 = call-dynamic "SetClassQueueMessage.vi"("ErrorIn(No Error)"=w307, "Menu déroulant"=w305, "DefaultDev.lvclass"=w309) -> ("sortie d'erreur"=w306:errorcluster, "DefaultDev.lvclass Out"=w308:refnum<class "AFG3102C.lvclass">)  [unwired: 7 in]
          }
          event "OutputImp": Value Change {
            n170 = event-data() -> ("NewVal"=w365:u16)  [unwired: 1 in, 5 out]
            n171 = local read "Con/Disc."() -> (w361:bool)
            n172 = property class="AFG3102C.lvclass"(reference=w363, error in=w364) -> (error out=w360:errorcluster, "Accessor:VisaRes"=w362:refnum<visa-resource-name>)  [unwired: 1 out]
            n173 = case shown="Vrai" w361 {
              tunnel: w365 -> [_ w376]
              tunnel: w362 -> [_ w377]
              tunnel: w360 -> [w366 w378]
              tunnel: [w366 w371] -> w359
              frame False {
              }
              frame True {
                w373 = u16 2 items=["Sine", "Square", "Pulse", "Ramp", "Noise", "DC", "Sin(x)/x", "Gaussian", "Lorentz", "Exponential Rise", "Exponential Decay", "Haversine"] ("Waveform Function (0: Sine)")
                w368 = u16 0 items=["Channel 1", "Channel2"] ("Channel (0: Channel 1)")
                n174 = local read "Custom Impedance"() -> (w367:dbl)
                n175 = call <userlib>:"Configure Output Impedance.vi"("Customized Impedance (50.0 Ohm)"=w367, "error in (no error)"=w378, "Impedance (0: 50 Ohm)"=w376, "Channel (0: Channel 1)"=w368, "VISA resource name"=w377) -> ("error out"=w372:errorcluster, "VISA resource name out"=w370:refnum<visa-resource-name>)  [unwired: 5 in]
                n176 = local read "HighLevel(V)"() -> (w375:dbl)
                n177 = local read "LowLevel(V)"() -> (w374:dbl)
                n178 = call <userlib>:"Configure Standard Waveform_Lev.vi"("VISA resource name"=w370, "Channel (0: Channel 1)"=w368, "Waveform Function (0: Sine)"=w373, "HighLevel (V)"=w375, "error in (no error)"=w372, "LowLevel (V)"=w374, "Phase Level (-1)"=0.0) -> ("error out"=w371:errorcluster)  [unwired: 7 in, 1 out]
              }
            }
          }
          event "OutputImpch2": Value Change {
            n179 = event-data() -> ("NewVal"=w385:u16)  [unwired: 1 in, 5 out]
            n180 = local read "Con/Disc."() -> (w381:bool)
            n181 = property class="AFG3102C.lvclass"(reference=w383, error in=w384) -> (error out=w380:errorcluster, "Accessor:VisaRes"=w382:refnum<visa-resource-name>)  [unwired: 1 out]
            n182 = case shown="Vrai" w381 {
              tunnel: w385 -> [_ w396]
              tunnel: w382 -> [_ w397]
              tunnel: w380 -> [w386 w398]
              tunnel: [w386 w391] -> w379
              frame False {
              }
              frame True {
                w393 = u16 2 items=["Sine", "Square", "Pulse", "Ramp", "Noise", "DC", "Sin(x)/x", "Gaussian", "Lorentz", "Exponential Rise", "Exponential Decay", "Haversine"] ("Waveform Function (0: Sine)")
                w388 = u16 1 items=["Channel 1", "Channel2"] ("Channel (0: Channel 1)")
                n183 = local read "Custom Impedance"() -> (w387:dbl)
                n184 = call <userlib>:"Configure Output Impedance.vi"("Customized Impedance (50.0 Ohm)"=w387, "error in (no error)"=w398, "Impedance (0: 50 Ohm)"=w396, "Channel (0: Channel 1)"=w388, "VISA resource name"=w397) -> ("error out"=w392:errorcluster, "VISA resource name out"=w390:refnum<visa-resource-name>)  [unwired: 5 in]
                n185 = local read "HighLevel(V)"() -> (w395:dbl)
                n186 = local read "LowLevel(V)"() -> (w394:dbl)
                n187 = call <userlib>:"Configure Standard Waveform_Lev.vi"("VISA resource name"=w390, "Channel (0: Channel 1)"=w388, "Waveform Function (0: Sine)"=w393, "HighLevel (V)"=w395, "error in (no error)"=w392, "LowLevel (V)"=w394, "Phase Level (-1)"=0.0) -> ("error out"=w391:errorcluster)  [unwired: 7 in, 1 out]
              }
            }
          }
          event "Con/Disc.": Value Change {
            n188 = event-data() -> ("NewVal"=w400:bool)  [unwired: 1 in, 5 out]
            n189 = property class="AFG3102C.lvclass"(reference=w405, error in=w403) -> (reference out=w404:refnum<class "AFG3102C.lvclass">, error out=w402:errorcluster, "Accessor:VisaRes"=w401:refnum<visa-resource-name>)
            n190 = case shown="Faux" w400 {
              tunnel: w402 -> [w408 w410]
              tunnel: w401 -> [w407 _]
              tunnel: [w406 w409] -> w399
              frame False {
                n191 = call <userlib>:"Close.vi"("error in (no error)"=w408, "VISA resource name"=w407) -> ("error out"=w406:errorcluster)  [unwired: 9 in]
              }
              frame True {
                n192 = property on="Init Program" class="Bool (strict)"(error in=w410, "Val(Sgnl)"=TRUE ("Valeur (Signalisation)")) -> (error out=w409:errorcluster)  [unwired: 1 in, 1 out]
              }
            }
          }
          event "Trigger Source", "ExtTrigger Slope", "IntTriggRate(s)": Value Change {
            n193 = event-data() -> ("NewVal"=w418:variant)  [unwired: 1 in, 5 out]
            n194 = local read "Con/Disc."() -> (w414:bool)
            n195 = property class="AFG3102C.lvclass"(reference=w416, error in=w417) -> (error out=w413:errorcluster, "Accessor:VisaRes"=w415:refnum<visa-resource-name>)  [unwired: 1 out]
            n196 = case shown="Vrai" w414 {
              tunnel: w418 -> [_ _]
              tunnel: w415 -> [_ w422]
              tunnel: w413 -> [w419 w421]
              tunnel: [w419 w423] -> w412
              frame False {
              }
              frame True {
                n197 = local read "IntTriggRate(s)"() -> (w420:dbl)
                n198 = local read "ExtTrigger Slope"() -> (w424:u16)
                n199 = local read "Trigger Source"() -> (w425:u16)
                n200 = call <userlib>:"Configure Trigger.vi"("External Trigger Slope (0: Positive)"=w424, "Internal Trigger Rate (500)"=w420, "error in (no error)"=w421, "Trigger Source (3:Internal)"=w425, "VISA resource name"=w422) -> ("error out"=w423:errorcluster)  [unwired: 5 in, 1 out]
              }
            }
          }
          event "PulseCount", "BurstDel_us", "PulseCount_ch2", "BurstDel_us_ch2": Value Change {
            n201 = event-data() -> ("NewVal"=w432:variant)  [unwired: 1 in, 5 out]
            n202 = local read "Con/Disc."() -> (w428:bool)
            n203 = property class="AFG3102C.lvclass"(reference=w430, error in=w431) -> (error out=w427:errorcluster, "Accessor:VisaRes"=w429:refnum<visa-resource-name>)  [unwired: 1 out]
            n204 = case shown="Vrai" w428 {
              tunnel: w432 -> [_ _]
              tunnel: w429 -> [_ w436]
              tunnel: w427 -> [w433 w437]
              tunnel: [w433 w435] -> w426
              frame False {
              }
              frame True {
                n205 = local read "Link Ch"() -> (w434:bool)
                n206 = case shown="Vrai" w434 {
                  tunnel: w437 -> [w452 w470]
                  tunnel: w436 -> [w449 w467]
                  tunnel: [w447 w464] -> w435
                  frame True {
                    w444 = u16 1 items=["Channel 1", "Channel2"] ("Channel (0: Channel 1)")
                    w445 = u16 0 items=["Triggered", "Gated"] ("Burst Mode (0: Triggered)")
                    w450 = u16 0 items=["Channel 1", "Channel2"] ("Channel (0: Channel 1)")
                    n207 = local read "BurstDel_us"() -> (w443:dbl)
                    n208 = local read "PulseCount"() -> (w439:i32)
                    n209 = local write "BurstDel_us_ch2"(w443) -> ()
                    n210 = expression code="1E-6*x"(w443) -> (w451:dbl)
                    n211 = call <userlib>:"Configure Burst.vi"("Busrt Delay  (0.0s)"=w451, "Burst Count (5)"=w439, "Enable Burst (T: Enable)"=TRUE ("Enable Burst"), "error in (no error)"=w452, "Burst Mode (0: Triggered)"=w445, "Channel (0: Channel 1)"=w450, "VISA resource name"=w449) -> ("error out"=w448:errorcluster, "VISA resource name out"=w446:refnum<visa-resource-name>)  [unwired: 3 in]
                    n212 = local read "PulsePeriod_us"() -> (w442:dbl)
                    n213 = call <userlib>:"Configure Burst.vi"("Burst Count (5)"=w439, "Enable Burst (T: Enable)"=TRUE, "error in (no error)"=w448, "Burst Mode (0: Triggered)"=w445, "Channel (0: Channel 1)"=w444, "VISA resource name"=w446) -> ("error out"=w447:errorcluster)  [unwired: 4 in, 1 out]
                    n214 = Multiply(x=w442, y=w439) -> (x*y=w441:dbl)
                    n215 = expression code="1E-6*x"(w441) -> (w440:dbl)
                    n216 = local write "PulseCount_ch2"(w439) -> ()
                    n217 = local write "AcqTime"(w440) -> ()
                  }
                  frame False {
                    w461 = u16 1 items=["Channel 1", "Channel2"] ("Channel (0: Channel 1)")
                    w462 = u16 0 items=["Triggered", "Gated"] ("Burst Mode (0: Triggered)")
                    w468 = u16 0 items=["Channel 1", "Channel2"] ("Channel (0: Channel 1)")
                    n218 = local read "BurstDel_us"() -> (w466:dbl)
                    n219 = local read "BurstDel_us_ch2"() -> (w460:dbl)
                    n220 = local read "PulseCount"() -> (w457:i32)
                    n221 = expression code="1E-6*x"(w466) -> (w469:dbl)
                    n222 = expression code="1E-6*x"(w460) -> (w459:dbl)
                    n223 = call <userlib>:"Configure Burst.vi"("Busrt Delay  (0.0s)"=w469, "Burst Count (5)"=w457, "Enable Burst (T: Enable)"=TRUE ("Enable Burst"), "error in (no error)"=w470, "Burst Mode (0: Triggered)"=w462, "Channel (0: Channel 1)"=w468, "VISA resource name"=w467) -> ("error out"=w465:errorcluster, "VISA resource name out"=w463:refnum<visa-resource-name>)  [unwired: 3 in]
                    n224 = local read "PulseCount_ch2"() -> (w454:i32)
                    n225 = local read "PulsePeriod_us"() -> (w458:dbl)
                    n226 = call <userlib>:"Configure Burst.vi"("Busrt Delay  (0.0s)"=w459, "Burst Count (5)"=w454, "error in (no error)"=w465, "Burst Mode (0: Triggered)"=w462, "Channel (0: Channel 1)"=w461, "VISA resource name"=w463) -> ("error out"=w464:errorcluster)  [unwired: 4 in, 1 out]
                    n227 = Multiply(x=w458, y=w457) -> (x*y=w456:dbl)
                    n228 = expression code="1E-6*x"(w456) -> (w455:dbl)
                    n229 = local write "AcqTime"(w455) -> ()
                  }
                }
              }
            }
          }
          event "BefDel_us", "PHighTime_us", "PLowTime_us", "AfterPulseDel(us)", "PHighTime_us_ch2", "PLowTime_us_ch2": Value Change {
            n230 = event-data() -> ()  [unwired: 1 in, 6 out]
            n231 = local read "Con/Disc."() -> (w474:bool)
            n232 = property class="AFG3102C.lvclass"(reference=w476, error in=w477) -> (error out=w473:errorcluster, "Accessor:VisaRes"=w475:refnum<visa-resource-name>)  [unwired: 1 out]
            n233 = case shown="Vrai" w474 {
              tunnel: w475 -> [_ w486]
              tunnel: w473 -> [w478 w488]
              tunnel: [w478 w487] -> w472
              frame False {
              }
              frame True {
                n234 = local read "Link Ch"() -> (w485:bool)
                n235 = local read "BefDel_us"() -> (w484:dbl)
                n236 = local read "PHighTime_us_ch2"() -> (w481:dbl)
                n237 = local read "PHighTime_us"() -> (w482:dbl)
                n238 = local read "PLowTime_us"() -> (w483:dbl)
                n239 = local read "PLowTime_us_ch2"() -> (w479:dbl)
                n240 = local read "AfterPulseDel(us)"() -> (w480:dbl)
                n241 = case shown="Vrai" w485 {
                  tunnel: w488 -> [w510 w540]
                  tunnel: [w497 w519] -> w487
                  tunnel: w486 -> [w509 w539]
                  tunnel: w484 -> [w507 w531]
                  tunnel: w482 -> [w504 w530]
                  tunnel: w483 -> [w505 _]
                  tunnel: w481 -> [w494 w532]
                  tunnel: w480 -> [_ w529]
                  tunnel: w479 -> [w493 _]
                  frame False {
                    w501 = 5e-09 ("Leading Edge Time (5.0E-8)")
                    w500 = u16 1 items=["Channel 1", "Channel2"] ("Channel (0: Channel 1)")
                    w511 = 5e-09 ("Leading Edge Time (5.0E-8)")
                    w508 = u16 0 items=["Channel 1", "Channel2"] ("Channel (0: Channel 1)")
                    n242 = Add(x=w504, y=w505) -> (x+y=w502:dbl)
                    n243 = local write "InitPulseHT_us"(w504) -> ()
                    n244 = expression code="1E-6*x"(w507) -> (w506:dbl)
                    n245 = expression code="1E-6*x"(w504) -> (w503:dbl)
                    n246 = local write "InitPulseLT_us"(w505) -> ()
                    n247 = expression code="1E-6*x"(w502) -> (w491:dbl)
                    n248 = local write "PulsePeriod_us"(w502) -> ()
                    n249 = call <userlib>:"Configure Pulse Waveform_Width.vi"("Width(s)"=w503, "Trailing Edge Time (5.0E-8)"=w511, "Delay (0 s)"=w506, "Leading Edge Time (5.0E-8)"=w511, "error in (no error)"=w510, "Period(s)"=w491, "Channel (0: Channel 1)"=w508, "VISA resource name"=w509) -> ("error out"=w499:errorcluster, "VISA resource name out"=w498:refnum<visa-resource-name>)  [unwired: 2 in]
                    n250 = local read "PulseCount"() -> (w490:i32)
                    n251 = local write "InitPulseHT_us_ch2"(w494) -> ()
                    n252 = local write "InitPulseLT_us_ch2"(w493) -> ()
                    n253 = Add(x=w494, y=w493) -> (x+y=w496:dbl)
                    n254 = expression code="1E-6*x"(w494) -> (w495:dbl)
                    n255 = expression code="1E-6*x"(w496) -> (w492:dbl)
                    n256 = local write "PulsePeriod_us_ch2"(w496) -> ()
                    n257 = Multiply(x=w491, y=w490) -> (x*y=w489:dbl)
                    n258 = call <userlib>:"Configure Pulse Waveform_Width.vi"("Width(s)"=w495, "Trailing Edge Time (5.0E-8)"=w501, "Leading Edge Time (5.0E-8)"=w501, "error in (no error)"=w499, "Period(s)"=w492, "Channel (0: Channel 1)"=w500, "VISA resource name"=w498) -> ("error out"=w497:errorcluster)  [unwired: 3 in, 1 out]
                    n259 = local write "AcqTime"(w489) -> ()
                  }
                  frame True {
                    w512 = 0.0 ("Busrt Delay  (0.0s)")
                    w534 = 5e-09 ("Leading Edge Time (5.0E-8)")
                    w513 = u16 0 items=["Triggered", "Gated"] ("Burst Mode (0: Triggered)")
                    w516 = TRUE ("Enable Burst")
                    w514 = u16 1 items=["Channel 1", "Channel2"] ("Channel (0: Channel 1)")
                    w541 = 5e-09 ("Leading Edge Time (5.0E-8)")
                    w525 = u16 0 items=["Channel 1", "Channel2"] ("Channel (0: Channel 1)")
                    n260 = Compound Arithmetic op=ADD(w531, w530, w529) -> (w527:dbl)
                    n261 = Compound Arithmetic op=ADD(w531, w532) -> (w523:dbl)
                    n262 = Compound Arithmetic op=ADD(w523, w529) -> (w528:dbl)
                    n263 = Compound Arithmetic op=ADD(w530, w528) -> (w524:dbl)
                    n264 = expression code="1E-6*x"(w530) -> (w535:dbl)
                    n265 = local write "InitPulseLT_us_ch2"(w527) -> ()
                    n266 = local write "PLowTime_us_ch2"(w527) -> ()
                    n267 = expression code="1E-6*x"(w524) -> (w522:dbl)
                    n268 = local write "PulsePeriod_us"(w524) -> ()
                    n269 = local write "PulsePeriod_us_ch2"(w524) -> ()
                    n270 = local write "InitPulseHT_us_ch2"(w532) -> ()
                    n271 = local write "PLowTime_us"(w528) -> ()
                    n272 = local write "InitPulseLT_us"(w528) -> ()
                    n273 = call <userlib>:"Configure Pulse Waveform_Width.vi"("Width(s)"=w535, "Trailing Edge Time (5.0E-8)"=w541, "Leading Edge Time (5.0E-8)"=w541, "error in (no error)"=w540, "Period(s)"=w522, "Channel (0: Channel 1)"=w525, "VISA resource name"=w539) -> ("error out"=w536:errorcluster, "VISA resource name out"=w526:refnum<visa-resource-name>)  [unwired: 3 in]
                    n274 = local read "PulseCount"() -> (w518:i32)
                    n275 = local write "BurstDel_us"(w523) -> ()
                    n276 = expression code="1E-6*x"(w523) -> (w517:dbl)
                    n277 = expression code="1E-6*x"(w532) -> (w533:dbl)
                    n278 = call <userlib>:"Configure Burst.vi"("Busrt Delay  (0.0s)"=w517, "Burst Count (5)"=w518, "Enable Burst (T: Enable)"=w516, "error in (no error)"=w536, "Burst Mode (0: Triggered)"=w513, "Channel (0: Channel 1)"=w525, "VISA resource name"=w526) -> ("error out"=w537:errorcluster, "VISA resource name out"=w538:refnum<visa-resource-name>)  [unwired: 3 in]
                    n279 = local write "PulseCount_ch2"(w518) -> ()
                    n280 = call <userlib>:"Configure Pulse Waveform_Width.vi"("Width(s)"=w533, "Trailing Edge Time (5.0E-8)"=w534, "Leading Edge Time (5.0E-8)"=w534, "error in (no error)"=w537, "Period(s)"=w522, "Channel (0: Channel 1)"=w514, "VISA resource name"=w538) -> ("error out"=w520:errorcluster, "VISA resource name out"=w515:refnum<visa-resource-name>)  [unwired: 3 in]
                    n281 = Multiply(x=w522, y=w518) -> (x*y=w521:dbl)
                    n282 = local write "BurstDel_us_ch2"(w512) -> ()
                    n283 = call <userlib>:"Configure Burst.vi"("Busrt Delay  (0.0s)"=w512, "Burst Count (5)"=w518, "Enable Burst (T: Enable)"=w516, "error in (no error)"=w520, "Burst Mode (0: Triggered)"=w513, "Channel (0: Channel 1)"=w514, "VISA resource name"=w515) -> ("error out"=w519:errorcluster)  [unwired: 3 in, 1 out]
                    n284 = local write "AcqTime"(w521) -> ()
                  }
                }
              }
            }
          }
          event "Link Ch": Value Change {
            n285 = event-data() -> ("NewVal"=w546:bool)  [unwired: 1 in]
            n286 = local read "Init Program"() -> (w544:bool)
            n287 = case shown="Faux" w544 {
              tunnel: [w557 w562] -> w552
              tunnel: w551 -> [w561 w562]
              frame False {
                n288 = local read "PHighTime_us"() -> (w560:dbl)
                n289 = local read "PulseCount"() -> (w559:i32)
                n290 = property on="PHighTime_us" class="NumNb (strict)"(error in=w561, "Val(Sgnl)"=w560) -> (error out=w558:errorcluster)  [unwired: 1 in, 1 out]
                n291 = property on="PulseCount" class="NumNb (strict)"(error in=w558, "Val(Sgnl)"=w559) -> (error out=w557:errorcluster)  [unwired: 1 in, 1 out]
              }
              frame True {
                n292 = local write "Init Program"(FALSE) -> ()
              }
            }
            n293 = control-ref of="PLowTime_us_ch2"() -> (w555:refnum<vi>)
            n294 = control-ref of="PulseCount_ch2"() -> (w554:refnum<vi>)
            n295 = control-ref of="PLowTime_us"() -> (w545:refnum<vi>)
            n296 = control-ref of="BurstDel_us"() -> (w543:refnum<vi>)
            n297 = control-ref of="BurstDel_us_ch2"() -> (w542:refnum<vi>)
            n298 = Build Array(w554, w555, w545, w543, w542) -> (w556:refnum<vi>[])
            n299 = Select(t=T3."DisAndGrayed" ("Énum"), s=w546, f=T3."Enable" ("Énum")) -> (s? t:f=w548:T3)
            n300 = call <userlib>:"SetCtrlPropGen.vi"("Error in"=w552, "Énum"=w548, "Controls"=w556) -> ("Error out"=w553:errorcluster)  [unwired: 3 in, 1 out]
          }
          event "Acq": Value Change {
            n301 = event-data() -> ("NewVal"=w565:bool)  [unwired: 1 in, 5 out]
            n302 = case shown="Faux" w565 {
              frame False {
                n303 = case shown="Vrai" FALSE {
                  frame False {
                  }
                  frame True {
                    n304 = local read "InitPulseHT_us"() -> (w570:dbl)
                    n305 = local read "InitPulseLT_us"() -> (w569:dbl)
                    n306 = local read "InitPulseHT_us_ch2"() -> (w567:dbl)
                    n307 = local read "InitPulseLT_us_ch2"() -> (w568:dbl)
                    n308 = local write "PHighTime_us"(w570) -> ()
                    n309 = local write "PHighTime_us_ch2"(w567) -> ()
                    n310 = local write "PLowTime_us"(w569) -> ()
                    n311 = local write "PLowTime_us_ch2"(w568) -> ()
                  }
                }
              }
              frame True {
              }
            }
          }
          event "LowLevel(V)": Value Change {
            n312 = event-data() -> ("NewVal"=w577:dbl)  [unwired: 1 in, 5 out]
            n313 = local read "Con/Disc."() -> (w573:bool)
            n314 = property class="AFG3102C.lvclass"(reference=w575, error in=w576) -> (error out=w572:errorcluster, "Accessor:VisaRes"=w574:refnum<visa-resource-name>)  [unwired: 1 out]
            n315 = case shown="Vrai" w573 {
              tunnel: w577 -> [_ w580]
              tunnel: w574 -> [_ w582]
              tunnel: w572 -> [w578 w583]
              tunnel: [w578 w584] -> w571
              frame False {
              }
              frame True {
                w579 = u16 1 items=["High", "Low"] ("Level (0:high)")
                w581 = u16 0 items=["Channel 1", "Channel2"] ("Channel (0: Channel 1)")
                n316 = call <userlib>:"Configure Level.vi"("VISA resource name"=w582, "Channel (0: Channel 1)"=w581, "Level (0:high)"=w579, "Level (V)"=w580, "error in (no error)"=w583) -> ("error out"=w584:errorcluster)  [unwired: 9 in, 1 out]
              }
            }
          }
          event "LowLevel(V)ch2": Value Change {
            n317 = event-data() -> ("NewVal"=w591:dbl)  [unwired: 1 in, 5 out]
            n318 = local read "Con/Disc."() -> (w587:bool)
            n319 = property class="AFG3102C.lvclass"(reference=w589, error in=w590) -> (error out=w586:errorcluster, "Accessor:VisaRes"=w588:refnum<visa-resource-name>)  [unwired: 1 out]
            n320 = case shown="Vrai" w587 {
              tunnel: w591 -> [_ w594]
              tunnel: w588 -> [_ w596]
              tunnel: w586 -> [w592 w597]
              tunnel: [w592 w598] -> w585
              frame False {
              }
              frame True {
                w593 = u16 1 items=["High", "Low"] ("Level (0:high)")
                w595 = u16 1 items=["Channel 1", "Channel2"] ("Channel (0: Channel 1)")
                n321 = call <userlib>:"Configure Level.vi"("VISA resource name"=w596, "Channel (0: Channel 1)"=w595, "Level (0:high)"=w593, "Level (V)"=w594, "error in (no error)"=w597) -> ("error out"=w598:errorcluster)  [unwired: 9 in, 1 out]
              }
            }
          }
          event "HighLevel(V)": Value Change {
            n322 = event-data() -> ("NewVal"=w605:dbl)  [unwired: 1 in, 5 out]
            n323 = local read "Con/Disc."() -> (w601:bool)
            n324 = property class="AFG3102C.lvclass"(reference=w603, error in=w604) -> (error out=w600:errorcluster, "Accessor:VisaRes"=w602:refnum<visa-resource-name>)  [unwired: 1 out]
            n325 = case shown="Vrai" w601 {
              tunnel: w605 -> [_ w608]
              tunnel: w602 -> [_ w610]
              tunnel: w600 -> [w606 w611]
              tunnel: [w606 w612] -> w599
              frame False {
              }
              frame True {
                w607 = u16 0 items=["High", "Low"] ("Level (0:high)")
                w609 = u16 0 items=["Channel 1", "Channel2"] ("Channel (0: Channel 1)")
                n326 = call <userlib>:"Configure Level.vi"("VISA resource name"=w610, "Channel (0: Channel 1)"=w609, "Level (0:high)"=w607, "Level (V)"=w608, "error in (no error)"=w611) -> ("error out"=w612:errorcluster)  [unwired: 9 in, 1 out]
              }
            }
          }
          event "HighLevel(V)ch2": Value Change {
            n327 = event-data() -> ("NewVal"=w619:dbl)  [unwired: 1 in, 5 out]
            n328 = local read "Con/Disc."() -> (w615:bool)
            n329 = property class="AFG3102C.lvclass"(reference=w617, error in=w618) -> (error out=w614:errorcluster, "Accessor:VisaRes"=w616:refnum<visa-resource-name>)  [unwired: 1 out]
            n330 = case shown="Vrai" w615 {
              tunnel: w619 -> [_ w622]
              tunnel: w616 -> [_ w624]
              tunnel: w614 -> [w620 w625]
              tunnel: [w620 w626] -> w613
              frame False {
              }
              frame True {
                w621 = u16 0 items=["High", "Low"] ("Level (0:high)")
                w623 = u16 1 items=["Channel 1", "Channel2"] ("Channel (0: Channel 1)")
                n331 = call <userlib>:"Configure Level.vi"("VISA resource name"=w624, "Channel (0: Channel 1)"=w623, "Level (0:high)"=w621, "Level (V)"=w622, "error in (no error)"=w625) -> ("error out"=w626:errorcluster)  [unwired: 9 in, 1 out]
              }
            }
          }
        }
        n332 = Or(x=w32, y="Stop") -> (x .or. y?=w30:bool)
      }
    }
    frame Error {
    }
  }
  "error out" <- w5
  "AFG3102C.lvclass Out" <- w3
